vi "Check Max Samples 5114.vi"(8 "error in (no error)":errorcluster, 9 "Encoder":i32, 10 "Max Samples":i32, 11 "Sample Count":i32) -> (0 "error out":errorcluster, 3 "Exceed Max?":bool)   [LabVIEW 2015, in "Tool Module.lvlib"]
doc: "<b>Note:</b> This VI was modified by the <b>Validate DQMH Module</b> tool to turn off automatic error handling."
uses:
  Tool Module.lvlib
  <vilib>/Utility/error.llb/Error Cluster From Error Code.vi
  <vilib>/ErrorRing/Error Ring.xnode
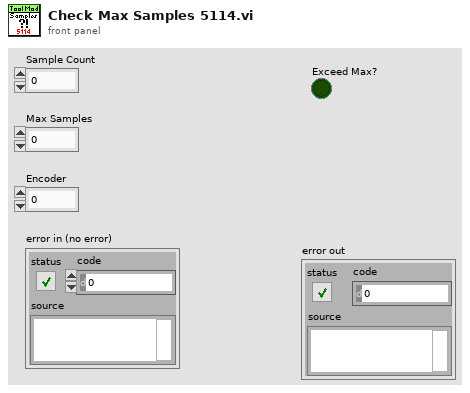
[diagram p1: front panel]
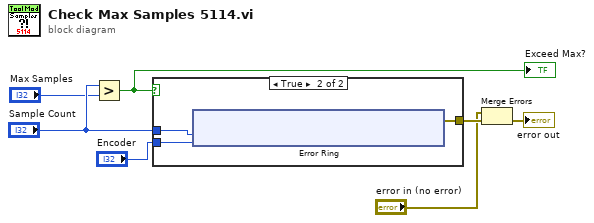
[diagram p0: block diagram]
diagram:
  n1 = Greater?(x="Sample Count", y="Max Samples") -> (0:w1:bool)
  "Exceed Max?" <- w1
  n2 = case shown="True" w1 {
    tunnel: "Encoder" -> [_ w10]
    tunnel: [_ w9] -> w6
    tunnel: "Sample Count" -> [_ w8]
    frame False {
    }
    frame True {
      n3 = xnode "Error Ring"("parameter 0"=w8, "parameter 1"=w10) -> ("error out"=w9:errorcluster)
    }
  }
  n4 = Merge Errors("error in (no error)", w6) -> (→"error out":errorcluster)
